vi "ConfigureMeasurementCamera.vi"(8 "error in":errorcluster, 9 "Set_Get":enum16{"Set", "Get"}(ring)=enum."Get", 11 "ConfigCamSet":T10(array[cluster])=[{"CameraIndex"=0, "SetAcquisitionMode"=enum."Reserved (0)", "SetOutputAmplifier"=enum."Standard EMCCD gain register", "SetExposureTime"=0.0, "SetNumberOfAccumulations"=0, "SetNumberOfKinetics"=0, "SetReadMode"=enum."Full Vertical Binning", "SetTriggerMode"=enum."Internal", "SetFastExternalTriggerModeOn"=FALSE, "SetFrameTransferMode"=enum."OFF", "SetSpoolMethod"=enum."32-bit", "SetFramebufferSize"=0, "SetCroppedMode"=FALSE, "SetExposure"=0.0, "SetAccumulate"=0.0, "SetKinetic"=0.0, "SetSpoolMode"=FALSE, "SetShutterTypeROI"=enum."TTL Low", "SetShutterModeROI"=enum."Open", "SetShutterClosingtimeROI"=0, "SetShutterOpeningtimeROI"=0, "SetAcquisitionModeROI"=enum."Run Till Abort", "SetReadModeROI"=enum."Image", "SetHorizontalBinningROI"=0, "SetVerticalBinningROI"=0, "SetExp.TimeROI"=0.0, "SetADChannelROI"=0, "typeSetHSSpeedsTypeROI"=enum."EM Amp", "SetHSSpeedsIndexROI"=0, "TriggermodeROI"=enum."Internal", "GetNumerVSSpeeds"=0, "GetTotalNumberOfPixelsROI"=0, "GetYDimensionROI"=0, "GetXDimensionROI"=0}]) -> (0 "error out":errorcluster, 3 "ConfigCamGet":T10(array[cluster]))   [LabVIEW 2011]
uses:
  Camera/lib/atmcd32d.llb/AcquisitionMode_mode typedef.ctl
  Camera/lib/atmcd32d.llb/OutputAmplifier_type typedef.ctl
  Camera/lib/atmcd32d.llb/ReadMode_mode typedef.ctl
  Camera/lib/atmcd32d.llb/DDGTriggerMode_mode typedef.ctl
  Camera/lib/atmcd32d.llb/Spool_method typedef.ctl
  Camera/lib/atmcd32d.llb/Shutter_type typedef.ctl
  Camera/lib/atmcd32d.llb/Shutter_mode typedef.ctl
  Camera/lib/atmcd32d.llb/HSSpeed_type typedef.ctl
  Camera/lib/atmcd32d.llb/TriggerMode_mode typedef.ctl
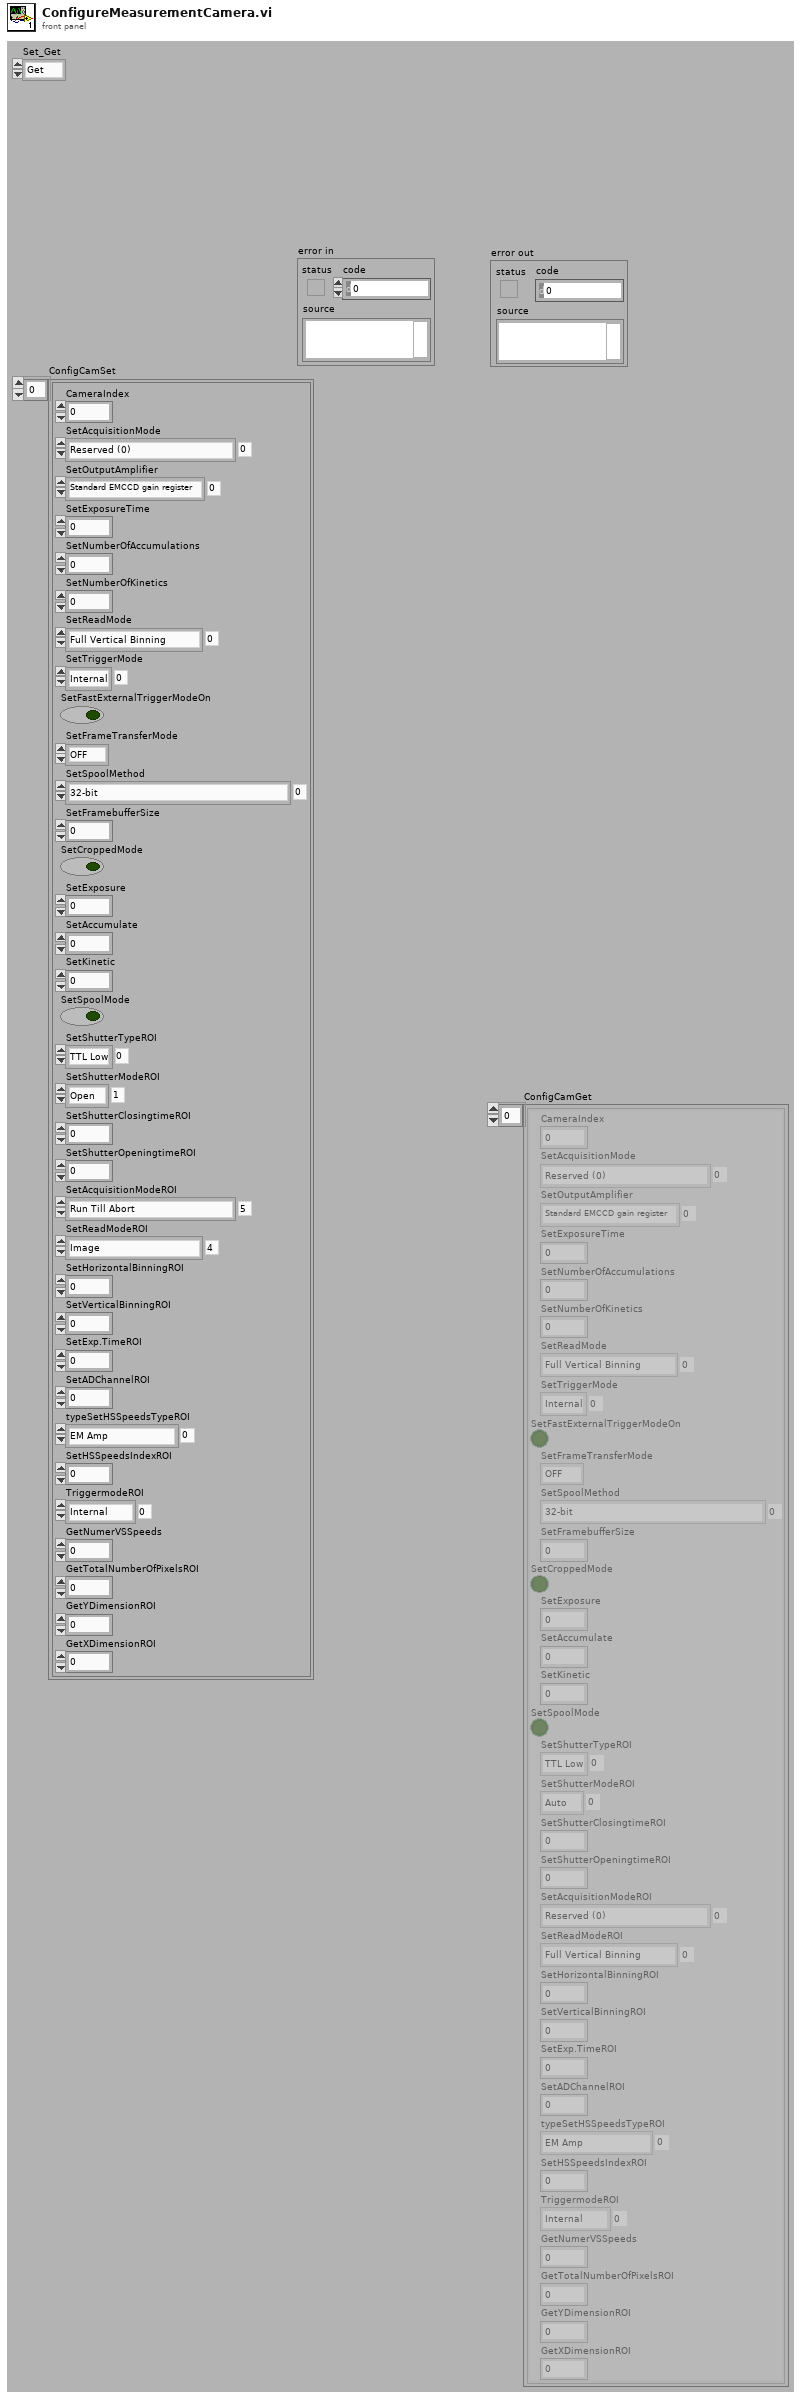
[diagram p1: front panel]
types:
  T1 = typedef "AcquisitionMode_mode typedef.ctl" = enum16{"Reserved (0)", "Single Scan", "Accumulate", "Kinetics", "Fast Kinetics", "Run Till Abort", "Reserved (6)", "Reserved (7)", "Reserved (8)", "Time Delayed Integration"}
  T2 = typedef "OutputAmplifier_type typedef.ctl" = enum16{"Standard EMCCD gain register", "Conventional CCD register"}
  T3 = typedef "ReadMode_mode typedef.ctl" = enum16{"Full Vertical Binning", "Multi-Track", "Random-Track", "Single-Track", "Image"}
  T4 = typedef "DDGTriggerMode_mode typedef.ctl" = enum16{"Internal", "External"}
  T5 = typedef "Spool_method typedef.ctl" = enum16{"32-bit", "Depends", "16-bit", "Multiple Directory", "Spool to RAM disk", "16-bit FITS", "SIF", "16-buit TIFF", "Multiple Directory Compressed"}
  T6 = typedef "Shutter_type typedef.ctl" = enum16{"TTL Low", "TTL High"}
  T7 = typedef "Shutter_mode typedef.ctl" = enum16{"Auto", "Open", "Close"}
  T8 = typedef "HSSpeed_type typedef.ctl" = enum16{"EM Amp", "Conventional Amp"}
  T9 = typedef "TriggerMode_mode typedef.ctl" = enum16{"Internal", "External", "N/A (2)", "N/A (3)", "N/A (4)", "N/A (5)", "External Start"}
  T10 = cluster{"CameraIndex":i32, "SetAcquisitionMode":T1, "SetOutputAmplifier":T2, "SetExposureTime":sgl, "SetNumberOfAccumulations":i32, "SetNumberOfKinetics":i32, "SetReadMode":T3, "SetTriggerMode":T4, "SetFastExternalTriggerModeOn":bool, "SetFrameTransferMode":enum16{"OFF", "ON"}, "SetSpoolMethod":T5, "SetFramebufferSize":i32, "SetCroppedMode":bool, "SetExposure":sgl, "SetAccumulate":sgl, "SetKinetic":sgl, "SetSpoolMode":bool, "SetShutterTypeROI":T6, "SetShutterModeROI":T7, "SetShutterClosingtimeROI":i32, "SetShutterOpeningtimeROI":i32, "SetAcquisitionModeROI":T1, "SetReadModeROI":T3, "SetHorizontalBinningROI":i32, "SetVerticalBinningROI":i32, "SetExp.TimeROI":sgl, "SetADChannelROI":i32, "typeSetHSSpeedsTypeROI":T8, "SetHSSpeedsIndexROI":i32, "TriggermodeROI":T9, "GetNumerVSSpeeds":i32, "GetTotalNumberOfPixelsROI":i32, "GetYDimensionROI":i32, "GetXDimensionROI":i32}[]
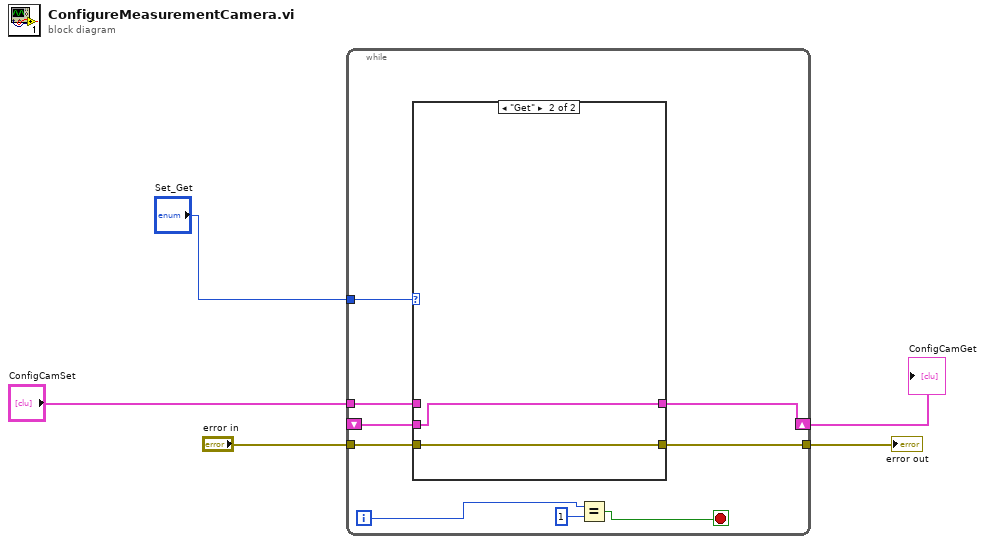
[diagram p0: block diagram]
diagram:
  n1 = while {
    tunnel: "Set_Get" -> [w14]
    tunnel: "error in" -> [w10]
    tunnel: [w9] -> w4
    tunnel: "ConfigCamSet" -> [w8]
    shift-right: [w7] -> w1
    shift-left: _ -> [w6]
    i -> [w11]
    stop <- w12 stop-if-true
    n2 = case shown="\"Get\"" w14 {
      tunnel: w10 -> [w16 w18]
      tunnel: [w16 w18] -> w9
      tunnel: w8 -> [w15 _]
      tunnel: [w15 w17] -> w7
      tunnel: w6 -> [_ w17]
      frame "Set", Default {
      }
      frame "Get" {
      }
    }
    n3 = Equal?(x=w11, y=1) -> (x = y?=w12:bool)
  }
  "error out" <- w4
  "ConfigCamGet" <- w1
